vi "Migrate G Plug-in.vi"() -> ()   [LabVIEW 2021]
uses:
  _Measurement Migrator/Migrator/Queue Driver/controls/Queue Operations.ctl
  _Measurement Migrator/Migrator/Migration Logic/controls/Multiple Migration/Multiple Migration Data Holder.ctl
  <vilib>/Utility/sysdir.llb/System Directory Type.ctl
  <vilib>/Utility/miscctls.llb/LVRowAndColumnUnsignedTypeDef.ctl
  <vilib>/Utility/miscctls.llb/LVRowAndColumnTypeDef.ctl
  _Measurement Migrator/Migrator/Migrator Reusables/controls/Dictionary States.ctl
  <vilib>/Utility/cursorutil.llb/Set Cursor (Icon Pict).vi
  _Measurement Migrator/Migrator/Queue Driver/Queue Driver.lvlib
  _Measurement Migrator/Migrator/Migration Logic/Migrator.lvlib
  _Measurement Migrator/Migrator/Path Functions/Path Functions.lvlib
  _Measurement Migrator/Migrator/Multiple Migrator/Multiple Migrator.lvlib
  _Measurement Migrator/Migrator/Migrator Reusables/Migrator Reusables.lvlib
  _Measurement Migrator/Migrator/G Plug-in Migrator/G Plug-in Migrator.lvlib
panel:
  out "error out":errorcluster
  in  "Tab Control":T1(tab)
  in  "Info":string
  in  "Select Measurement":path
  out "Warning":bool=TRUE caption="Warning:\nSelected folder contains invalid folder/file names"
  in  "Populate measurements":bool
  in  "Select Project":path
  in  "Select all":bool
  in  "Back to Home":bool
  in  "List Plug-ins":bool
  in  "Select Measurements":string(tree)
  out "Selection warning":string="Atleast one measurement should be selected"
  out "Plug-in info":string="* Rename the Plug-in if required"
  out "Plug-in warning":string="Warning:\n1. Measurement plug-in name must be unique \n2. Plugin name cannot contain any of the following characters:\n         \\ / : * ? \" < > |"
  in  "Start Migration":bool
  in  "Back to Select":bool
  in  "List of Selected Measurements":i32(listbox)
  in  "Measurement Count":i32(slide)=6 caption="Migrating 2 of 2 measurement(s)" scale=0.0..100.0
  in  "Progress":i32(slide)=9 caption="Saving the project files..." scale=0.0..15.0
  in  "Review":bool
  in  "Migration Status":i32(listbox)
  in  "Back to Status":bool
  in  "Select Plug-in":string(combo) caption="Select Measurement plug-in to review"
  in  "Start Next":bool
  out "Launch Type Spec":string
  out "Launch Logic":string
  out "Launch UI":string
  # "* Project in which the measurement plug-in will be created"
  # "* Select a measurement vi or a folder containing measurements"
  # ".lvproj"
  # "Select the measurements to migrate"
  # "Review the Measurement:\n1. Review the Measurement UI. Click here to launch.\n2. Review the Measurement Logic VI. Click here to launch.\n3. Review the Type Specialization VI. Click here to launch."
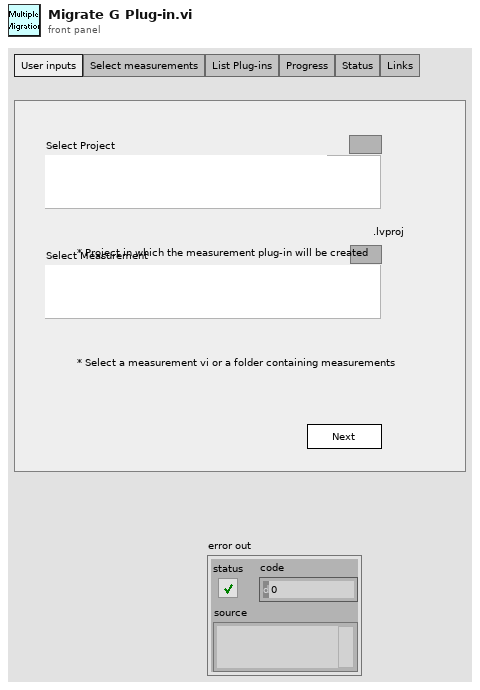
[diagram p1: front panel]
types:
  T1 = enum32{"User inputs", "Select measurements", "List Plug-ins", "Progress", "Status", "Links"}
  T2 = typedef "Queue Driver.lvlib/Queue Operations.ctl" = enum16{"Create Q", "Enqueue", "Enqueue N", "Dequeue", "Flush", "Release"}
  T3 = typedef "Migrator.lvlib/Multiple Migration Data Holder.ctl" = cluster{"Tree Reference":refnum<vi>, "LabVIEW Version":string, "Project path":path, "Create new project?":bool, "Measurement file/folder path":path, "Measurement folder selected?":bool, "Project warning":string, "Measurement warning":string, "Next clicked?":bool, "Measurement path changed?":bool, "Select all":bool, "Measurement folder Tags":string[], "Measurement file Tags":string[], "Selected cell Tag":string, "Measurement Plug-ins":string[][], "Measurement File Paths":path[], "Plugin Migration Value":i32, "Migration Count":i32, "Instrument containing subVIs":path[][], "Progress per measurement":i32, "Measurement Progress":i32, "Migration Status":string[][], "Selected Measurement":string[]}
  T4 = enum8{"Enabled", "Disabled", "Disabled and Grayed Out"}
  T5 = typedef "LVRowAndColumnUnsignedTypeDef.ctl" = cluster{"Row":u32, "Column":u32}
  T6 = typedef "LVRowAndColumnTypeDef.ctl" = cluster{"Row":i32, "Column":i32}
  T7 = typedef "Migrator Reusables.lvlib/Dictionary States.ctl" = enum16{"Set", "Get", "Delete", "Delete All"}
  T8 = typedef "System Directory Type.ctl" = i32
  T9 = typedef "LVPoint32TypeDef.ctl" = cluster{"Horizontal":i32, "Vertical":i32}
  T10 = typedef "Migrator.lvlib/Tree Items.ctl" = cluster{"Item name":string, "Indent":i32, "Tag":string}
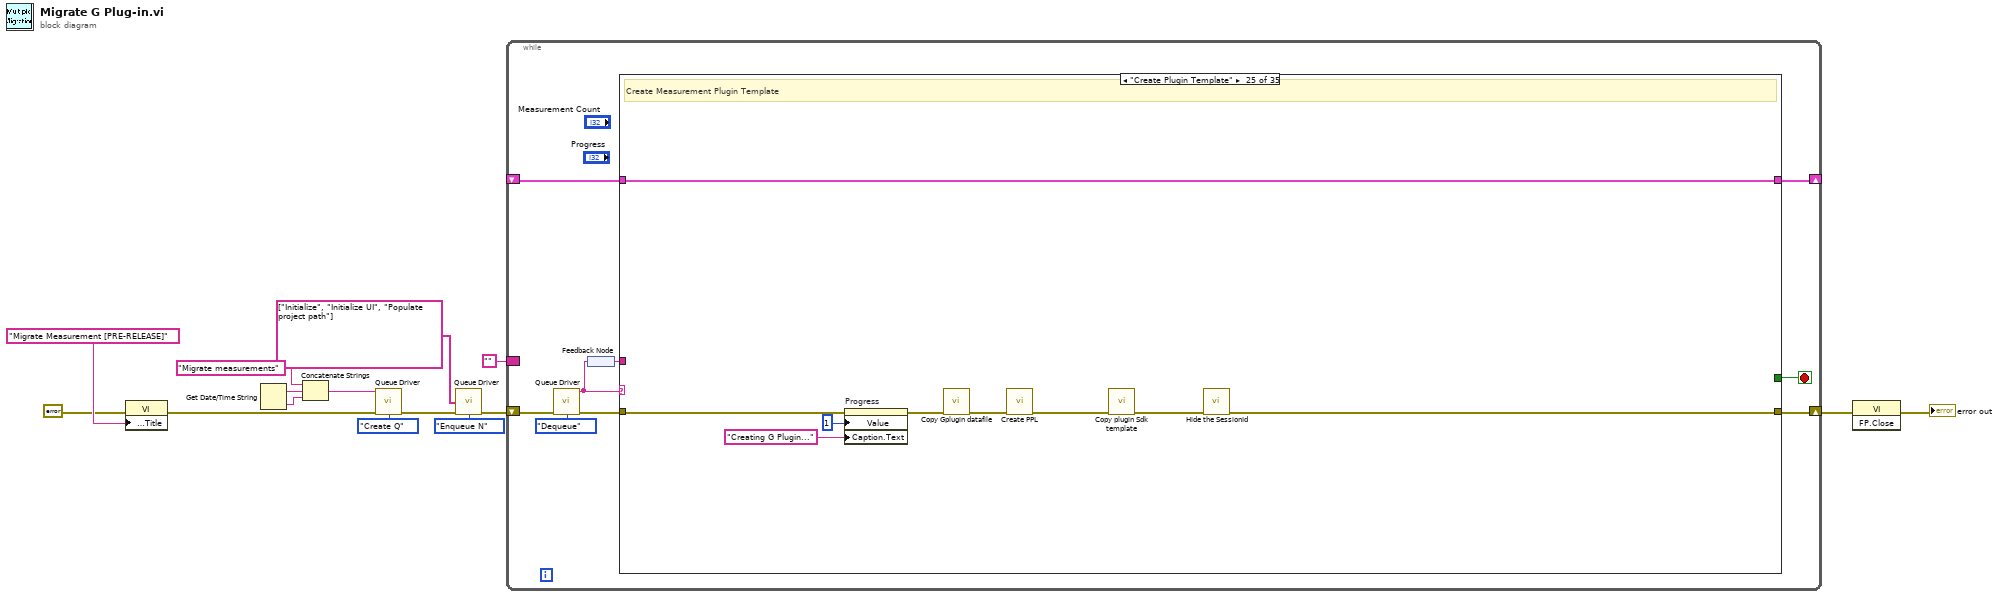
[diagram p0: block diagram]
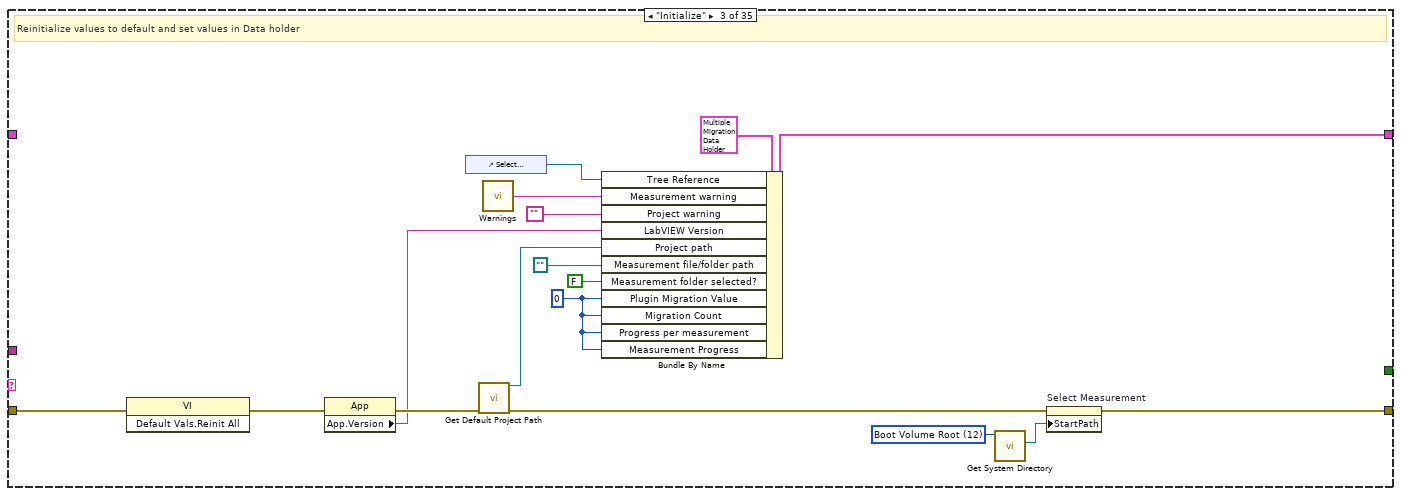
[diagram p4: hidden frame]
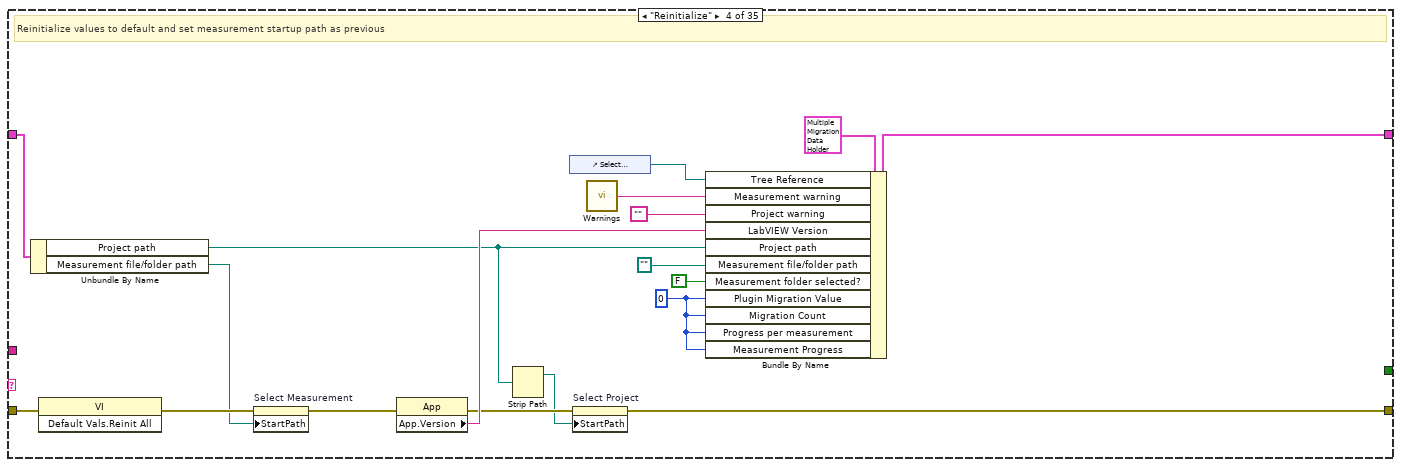
[diagram p5: hidden frame]
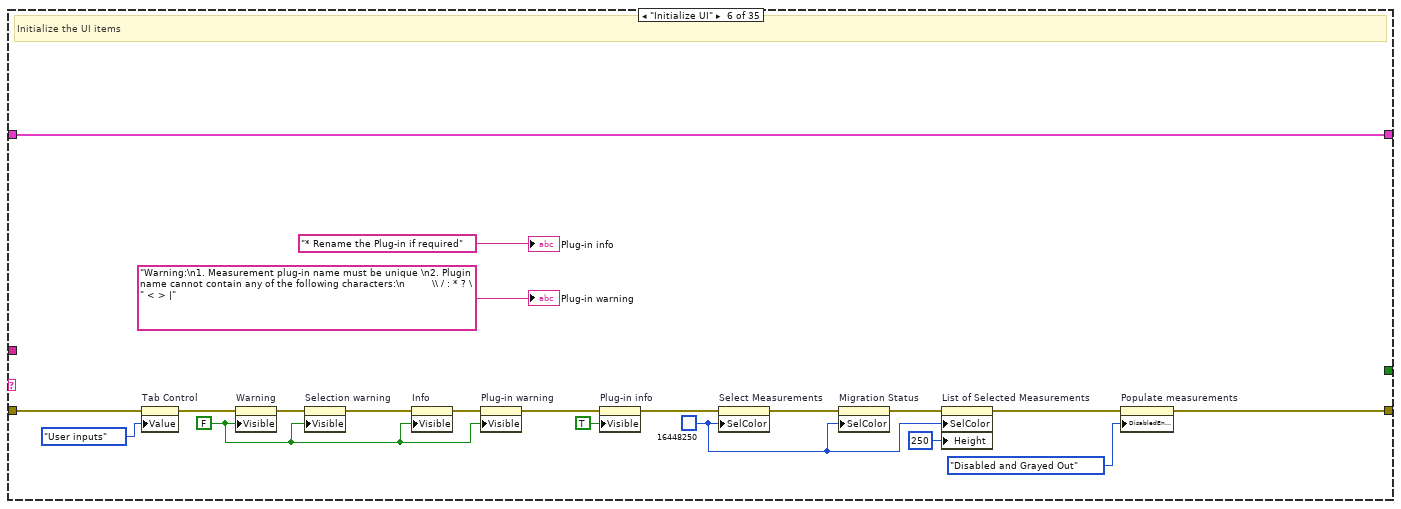
[diagram p7: hidden frame]
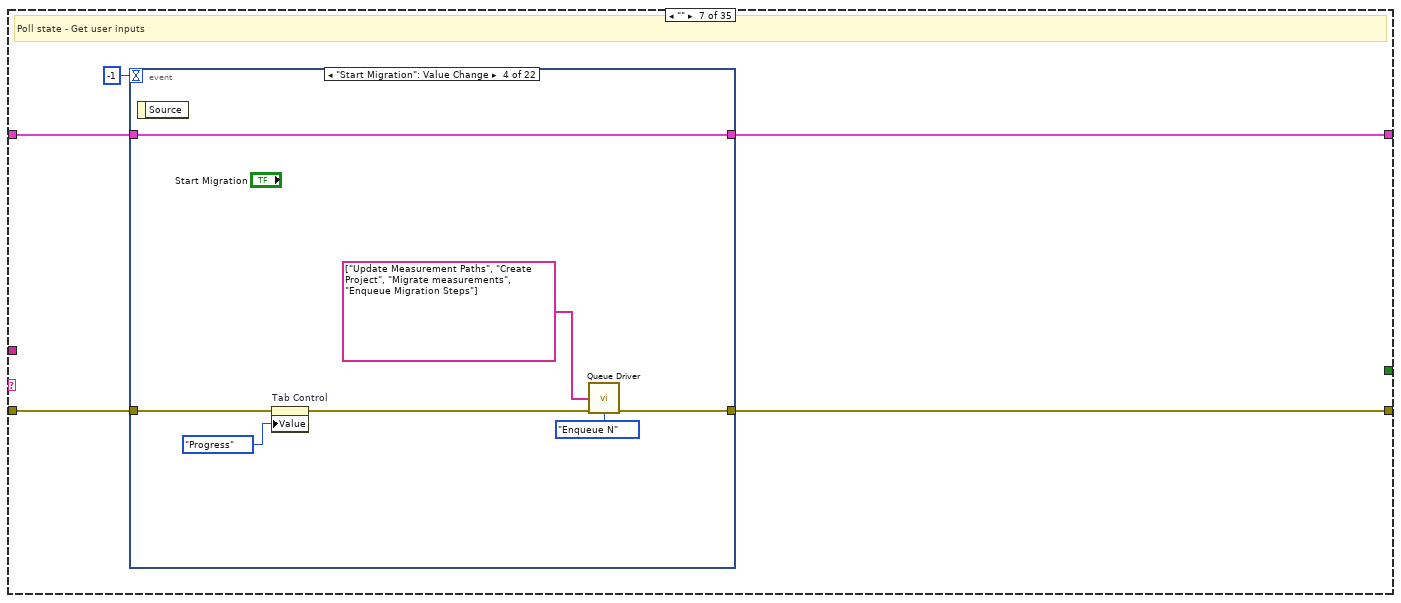
[diagram p8: hidden frame]
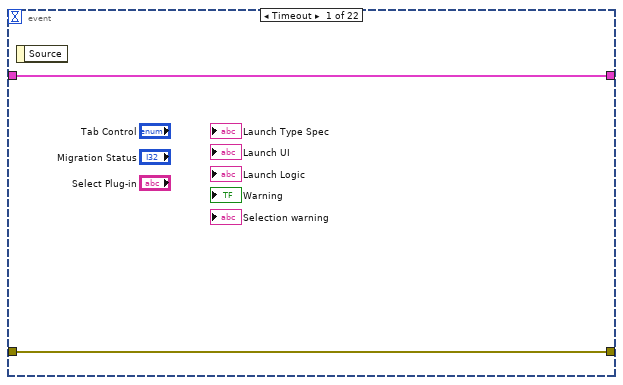
[diagram p9: hidden frame]
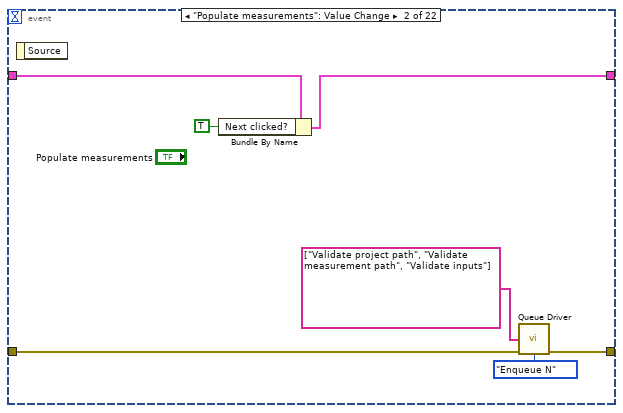
[diagram p10: hidden frame]
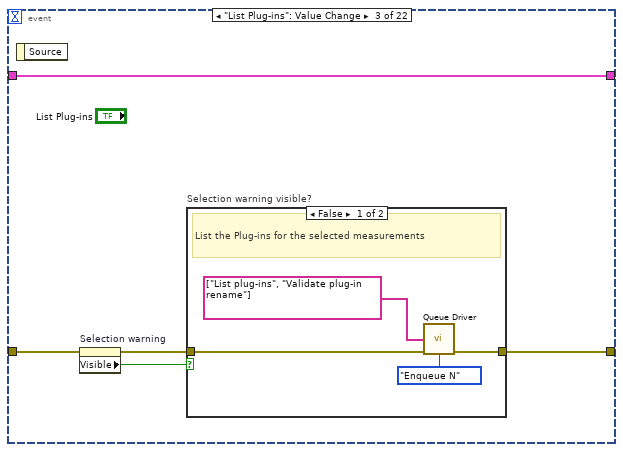
[diagram p11: hidden frame]
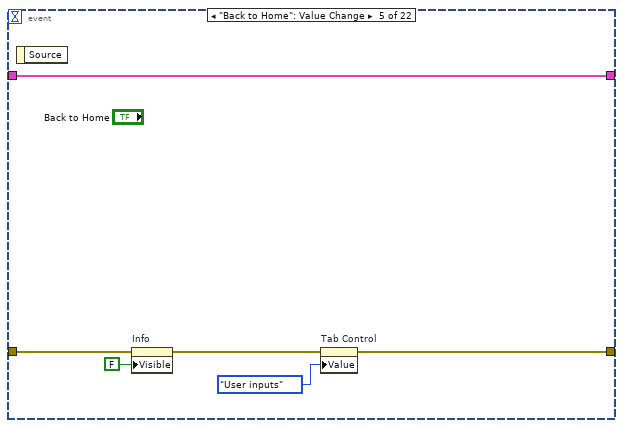
[diagram p13: hidden frame]
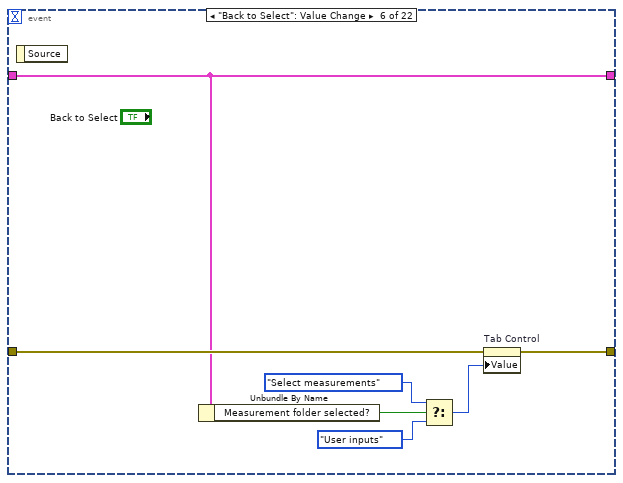
[diagram p14: hidden frame]
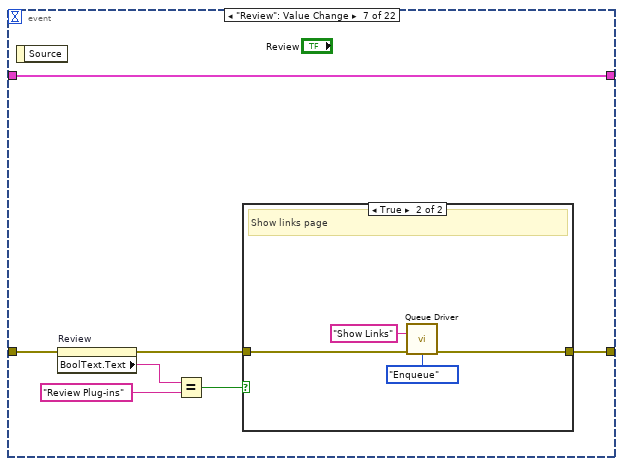
[diagram p15: hidden frame]
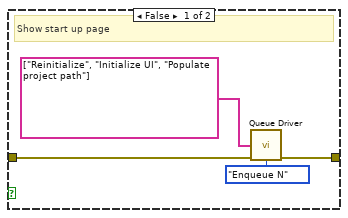
[diagram p16: hidden frame]
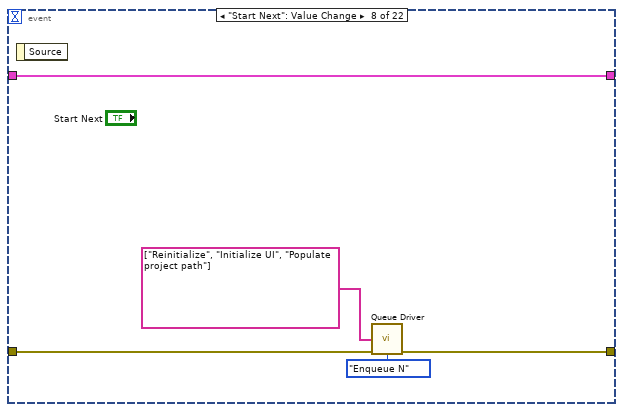
[diagram p17: hidden frame]
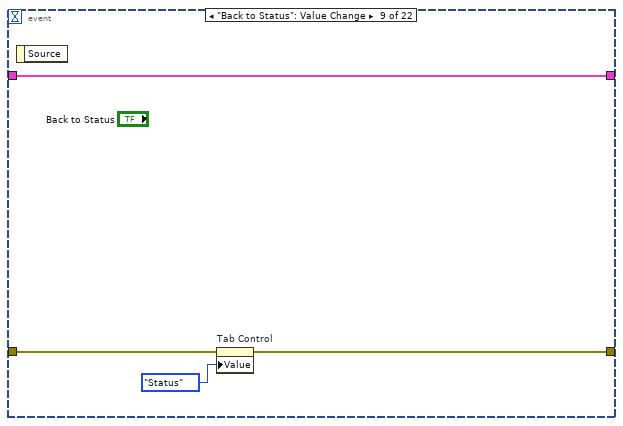
[diagram p18: hidden frame]
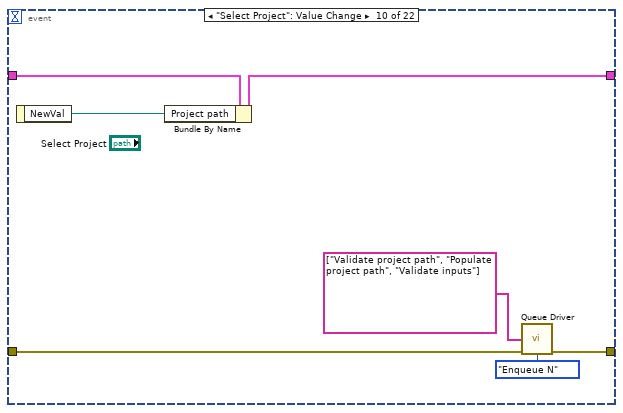
[diagram p19: hidden frame]
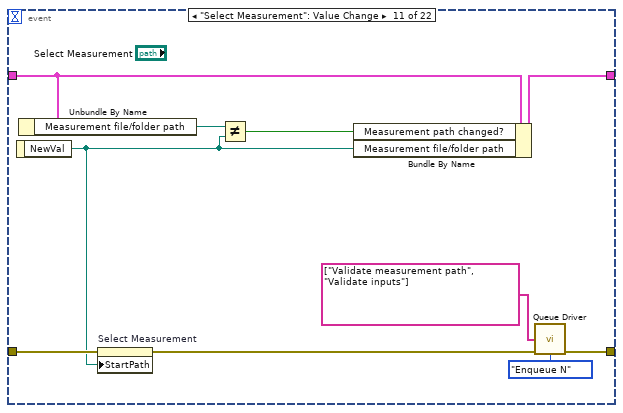
[diagram p20: hidden frame]
diagram:
  n1 = property class="VI"(error in=errorcluster {"status"=FALSE, "code"=0, "source"=""} ("error in (no error)"), "Front Panel.Title"="Migrate Measurement [PRE-RELEASE]" ("Front Panel Window:Title")) -> (error out=w1:errorcluster)  [unwired: 1 in, 1 out]
  n2 = Get Date/Time String() -> (date string=w12:string, time string=w11:string)  [unwired: 3 in]
  n3 = Concatenate Strings("Migrate measurements" ("string"), w12, w11) -> (w7:string)
  n4 = call "Queue Driver.vi"("Name"=w7, "error in (no error)"=w1, "Q Operations"=Queue_Operations."Create Q") -> ("error out"=w15:errorcluster)  [unwired: 11 in, 1 out]
  n5 = call "Queue Driver.vi"("States[]"=string[] ["Initialize", "Initialize UI", "Populate project path"], "error in (no error)"=w15, "Q Operations"=Queue_Operations."Enqueue N") -> ("error out"=w10:errorcluster)  [unwired: 11 in, 1 out]
  n6 = while {
    shift-right: [w23] -> w6
    shift-left: w10 -> [w24]
    shift-right: [w20] -> _
    shift-left: _ -> [w19]
    border: "" -> [_]
    stop <- w18 stop-if-true
    n7 = call "Queue Driver.vi"("error in (no error)"=w24, "Q Operations"=Queue_Operations."Dequeue") -> ("Dequeued State"=w17:string, "error out"=w22:errorcluster)  [unwired: 12 in]
    n8 = feedback #1() -> (w16:string)
    n9 = feedback-in #1(w17) -> ()
    n10 = case shown="\"Create Plugin Template\"" w17 {
      tunnel: w22 -> [w25 w28 w45 w63 w65 w85 w90 w265 w277 w288 w307 w331 w376 w393 w446 w471 w492 w549 w559 w566 w586 w596 w615 w632 w658 w662 w668 w690 w711 w723 w765 w774 w783 w804 w816]
      tunnel: [w25 w28 w34 w48 w65 w76 w89 w267 w277 w280 w306 w330 w376 w388 w434 w454 w479 w539 w559 w561 w583 w599 w614 w631 w653 w663 w672 w694 w711 w722 w762 w774 w780 w804 w806] -> w23
      tunnel: [w26 w27 w44 w62 w64 w81 w86 w266 w278 w283 w300 w318 w377 w394 w437 w469 w476 w544 w558 w578 w594 w608 w618 w651 w660 w666 w673 w695 w712 w727 w764 w775 w785 w805 w814] -> w20
      tunnel: w19 -> [w26 w27 _ w51 w64 w81 w87 w266 w278 w284 w302 w329 w377 w395 w438 w470 w477 w545 w558 w579 w594 w607 w618 w651 w660 w666 w674 w696 w712 w728 w764 w775 w785 w805 w814]
      tunnel: [_ _ _ _ _ _ _ _ _ _ _ _ _ _ _ _ _ _ _ _ _ _ _ _ _ _ _ _ _ _ _ _ _ _ TRUE] -> w18
      tunnel: w16 -> [_ _ _ _ _ _ _ _ _ _ _ _ _ _ _ _ _ _ _ _ _ _ _ _ _ _ _ _ _ _ _ _ w776 _ _]
      frame Default {
        # "Default case"
      }
      frame "/**********INITIALIZE**********/" {
      }
      frame "Initialize" {
        w29 = 0 ("Plugin Migration Value")
        w33 = T8 12 items=["User Home"=0, "User Desktop"=1, "User Documents"=2, "User Application Data"=3, "User Preferences"=4, "User Temporary"=5, "Public Documents"=6, "Public Application Data"=7, "Public Preferences"=8, "Public Cache"=13, "System Core Libraries"=9, "System Installed Libraries"=10, "Application Files"=11, "Boot Volume Root"=12] ("system directory type")
        # "Reinitialize values to default and set values in Data holder"
        n11 = invoke class="VI" method="Default Vals.Reinit All"(error in=w45) -> (error out=w42:errorcluster)  [unwired: 2 in, 2 out]
        n12 = property class="App"(error in=w42) -> (error out=w41:errorcluster, "App.Version"=w40:string)  [unwired: 1 in, 1 out]
        n13 = control-ref of="Select Measurements"() -> (w37:refnum<vi>)
        n14 = call "Get Default Project Path.vi"("error in"=w41) -> ("Project Path"=w43:path, "error out"=w35:errorcluster)  [unwired: 13 in]
        n15 = call "Warnings.vi"() -> ("Invalid measurement path"=w36:string)  [unwired: 8 in, 7 out]
        n16 = Bundle By Name(cluster=T3 {"Tree Reference"=refnum, "LabVIEW Version"="", "Project path"=path "", "Create new project?"=FALSE, "Measurement file/folder path"=path "", "Measurement folder selected?"=FALSE, "Project warning"="", "Measurement warning"="", "Next clicked?"=FALSE, "Measurement path changed?"=FALSE, "Select all"=FALSE, "Measurement folder Tags"=[], "Measurement file Tags"=[], "Selected cell Tag"="", "Measurement Plug-ins"=[], "Measurement File Paths"=[], "Plugin Migration Value"=0, "Migration Count"=0, "Instrument containing subVIs"=[], "Progress per measurement"=0, "Measurement Progress"=0, "Migration Status"=[], "Selected Measurement"=[]}, "Tree Reference"=w37, "Measurement warning"=w36, "Project warning"="", "LabVIEW Version"=w40, "Project path"=w43, "Measurement file/folder path"=path "", "Measurement folder selected?"=FALSE, "Plugin Migration Value"=w29, "Migration Count"=w29, "Progress per measurement"=w29, "Measurement Progress"=w29) -> (w44:T3)
        n17 = call <vilib>:"Get System Directory.vi"("system directory type"=w33) -> ("system directory"=w32:path)  [unwired: 10 in]
        n18 = property on="Select Measurement" class="Path"(error in=w35, "StartPath"=w32) -> (error out=w34:errorcluster)  [unwired: 1 in, 1 out]
      }
      frame "Reinitialize" {
        w54 = 0 ("Plugin Migration Value")
        # "Reinitialize values to default and set measurement startup path as previous"
        n19 = Unbundle By Name(w51) -> ("Project path"=w47:path, "Measurement file/folder path"=w50:path)
        n20 = invoke class="VI" method="Default Vals.Reinit All"(error in=w63) -> (error out=w53:errorcluster)  [unwired: 2 in, 2 out]
        n21 = property on="Select Measurement" class="Path"(error in=w53, "StartPath"=w50) -> (error out=w52:errorcluster)  [unwired: 1 in, 1 out]
        n22 = property class="App"(error in=w52) -> (error out=w49:errorcluster, "App.Version"=w61:string)  [unwired: 1 in, 1 out]
        n23 = Strip Path(path=w47) -> (stripped path=w46:path)  [unwired: 1 out]
        n24 = control-ref of="Select Measurements"() -> (w58:refnum<vi>)
        n25 = property on="Select Project" class="Path"(error in=w49, "StartPath"=w46) -> (error out=w48:errorcluster)  [unwired: 1 in, 1 out]
        n26 = call "Warnings.vi"() -> ("Invalid measurement path"=w57:string)  [unwired: 8 in, 7 out]
        n27 = Bundle By Name(cluster=T3 {"Tree Reference"=refnum, "LabVIEW Version"="", "Project path"=path "", "Create new project?"=FALSE, "Measurement file/folder path"=path "", "Measurement folder selected?"=FALSE, "Project warning"="", "Measurement warning"="", "Next clicked?"=FALSE, "Measurement path changed?"=FALSE, "Select all"=FALSE, "Measurement folder Tags"=[], "Measurement file Tags"=[], "Selected cell Tag"="", "Measurement Plug-ins"=[], "Measurement File Paths"=[], "Plugin Migration Value"=0, "Migration Count"=0, "Instrument containing subVIs"=[], "Progress per measurement"=0, "Measurement Progress"=0, "Migration Status"=[], "Selected Measurement"=[]}, "Tree Reference"=w58, "Measurement warning"=w57, "Project warning"="", "LabVIEW Version"=w61, "Project path"=w47, "Measurement file/folder path"=path "", "Measurement folder selected?"=FALSE, "Plugin Migration Value"=w54, "Migration Count"=w54, "Progress per measurement"=w54, "Measurement Progress"=w54) -> (w62:T3)
      }
      frame "/**********FP RELATED**********/" {
      }
      frame "Initialize UI" {
        w70 = FALSE ("Visible")
        w78 = u32 16448250 ("Selection Color")
        # "Initialize the UI items"
        n28 = property on="Tab Control" class="TabCtl (strict)"(error in=w85, "Value"=T1."User inputs" ("Tab Control")) -> (error out=w80:errorcluster)  [unwired: 1 in, 1 out]
        n29 = property on="Warning" class="Bool"(error in=w80, "Visible"=w70) -> (error out=w79:errorcluster)  [unwired: 1 in, 1 out]
        n30 = property on="Selection warning" class="Str"(error in=w79, "Visible"=w70) -> (error out=w74:errorcluster)  [unwired: 1 in, 1 out]
        n31 = property on="Info" class="Str"(error in=w74, "Visible"=w70) -> (error out=w73:errorcluster)  [unwired: 1 in, 1 out]
        n32 = property on="Plug-in warning" class="Str"(error in=w73, "Visible"=w70) -> (error out=w69:errorcluster)  [unwired: 1 in, 1 out]
        n33 = property on="Plug-in info" class="Str"(error in=w69, "Visible"=TRUE) -> (error out=w68:errorcluster)  [unwired: 1 in, 1 out]
        n34 = property on="Select Measurements" class="Tree (strict)"(error in=w68, "SelColor"=w78) -> (error out=w83:errorcluster)  [unwired: 1 in, 1 out]
        n35 = property on="Migration Status" class="MCListbox (strict)"(error in=w83, "SelColor"=w78) -> (error out=w82:errorcluster)  [unwired: 1 in, 1 out]
        n36 = property on="List of Selected Measurements" class="MCListbox (strict)"(error in=w82, "SelColor"=w78, "Height"=u32 250 ("Size:Height")) -> (error out=w77:errorcluster)  [unwired: 1 in, 1 out]
        n37 = property on="Populate measurements" class="Bool"(error in=w77, "DisabledEnum"=T4."Disabled and Grayed Out" ("Disabled")) -> (error out=w76:errorcluster)  [unwired: 1 in, 1 out]
        "Plug-in warning" <- "Warning:\n1. Measurement plug-in name must be unique \n2. Plugin name cannot contain any of the following characters:\n         \\ / : * ? \" < > |" ("f")
        "Plug-in info" <- "* Rename the Plug-in if required" ("Plug-in warning")
      }
      frame "" {
        # "Poll state - Get user inputs"
        n38 = event shown="[3] \"Start Migration\": Value Change" {
          selector: _ -> [_ _ _ _ _ _ _ _ _ _ _ _ _ _ _ _ _ _ _ _ _ _]
          dyn-events: _ -> [_ _ _ _ _ _ _ _ _ _ _ _ _ _ _ _ _ _ _ _ _ _]
          timeout: -1 -> [_ _ _ _ _ _ _ _ _ _ _ _ _ _ _ _ _ _ _ _ _ _]
          tunnel: w90 -> [w92 w99 w102 w116 w119 w129 w133 w146 w153 w160 w166 w174 w185 w192 w205 w212 w215 w219 w225 w235 w247 w259]
          tunnel: [w92 w98 w103 w112 w122 w128 w135 w147 w152 w159 w169 w173 w180 w191 w203 w213 w216 w220 w227 w238 w249 w258] -> w89
          tunnel: w87 -> [w91 w95 w104 w113 w120 w127 w136 w149 w150 w157 w164 w177 w184 w193 w206 w214 w218 w222 w228 w239 w250 w260]
          tunnel: [w91 w94 w104 w113 w120 w127 w136 w149 w150 w156 w170 w176 w183 w193 w206 w214 w218 w222 w228 w239 w250 w260] -> w86
          event Timeout {
            # "Timeout"
            n39 = event-data() -> ()  [unwired: 1 in, 1 out]
          }
          event "Populate measurements": Value Change {
            n40 = event-data() -> ()  [unwired: 1 in, 1 out]
            n41 = Bundle By Name(cluster=w95, "Next clicked?"=TRUE) -> (w94:T3)
            n42 = call "Queue Driver.vi"("States[]"=string[] ["Validate project path", "Validate measurement path", "Validate inputs"], "error in (no error)"=w99, "Q Operations"=Queue_Operations."Enqueue N") -> ("error out"=w98:errorcluster)  [unwired: 11 in, 1 out]
          }
          event "List Plug-ins": Value Change {
            n43 = event-data() -> ()  [unwired: 1 in, 1 out]
            n44 = property on="Selection warning" class="Str"(error in=w102) -> (error out=w101:errorcluster, "Visible"=w100:bool)  [unwired: 1 in, 1 out]
            n45 = case "Selection warning visible?" shown="False" w100 {
              tunnel: w101 -> [w108 w109]
              tunnel: [w107 w109] -> w103
              frame False {
                # "List the Plug-ins for the selected measurements"
                n46 = call "Queue Driver.vi"("States[]"=string[] ["List plug-ins", "Validate plug-in rename"], "error in (no error)"=w108, "Q Operations"=Queue_Operations."Enqueue N") -> ("error out"=w107:errorcluster)  [unwired: 11 in, 1 out]
              }
              frame True {
                # "Pass"
              }
            }
          }
          event "Start Migration": Value Change {
            n47 = event-data() -> ()  [unwired: 1 in, 1 out]
            n48 = property on="Tab Control" class="TabCtl (strict)"(error in=w116, "Value"=T1."Progress" ("Tab Control")) -> (error out=w115:errorcluster)  [unwired: 1 in, 1 out]
            n49 = call "Queue Driver.vi"("States[]"=string[] ["Update Measurement Paths", "Create Project", "Migrate measurements", "Enqueue Migration Steps"], "error in (no error)"=w115, "Q Operations"=Queue_Operations."Enqueue N") -> ("error out"=w112:errorcluster)  [unwired: 11 in, 1 out]
          }
          event "Back to Home": Value Change {
            n50 = event-data() -> ()  [unwired: 1 in, 1 out]
            n51 = property on="Info" class="Str"(error in=w119, "Visible"=FALSE) -> (error out=w118:errorcluster)  [unwired: 1 in, 1 out]
            n52 = property on="Tab Control" class="TabCtl (strict)"(error in=w118, "Value"=T1."User inputs" ("Tab Control")) -> (error out=w122:errorcluster)  [unwired: 1 in, 1 out]
          }
          event "Back to Select": Value Change {
            n53 = event-data() -> ()  [unwired: 1 in, 1 out]
            n54 = Unbundle By Name(w127) -> ("Measurement folder selected?"=w126:bool)
            n55 = Select(t=T1."Select measurements" ("Tab Control"), s=w126, f=T1."User inputs" ("Tab Control")) -> (s? t:f=w123:T1)
            n56 = property on="Tab Control" class="TabCtl (strict)"(error in=w129, "Value"=w123) -> (error out=w128:errorcluster)  [unwired: 1 in, 1 out]
          }
          event "Review": Value Change {
            n57 = event-data() -> ()  [unwired: 1 in, 1 out]
            n58 = property on="Review" class="Bool"(error in=w133) -> (error out=w134:errorcluster, "BoolText.Text"=w132:string)  [unwired: 1 in, 1 out]
            n59 = Equal?(x=w132, y="Review Plug-ins") -> (x = y?=w130:bool)
            n60 = case shown="True" w130 {
              tunnel: [w138 w144] -> w135
              tunnel: w134 -> [w137 w141]
              frame False {
                # "Show start up page"
                n61 = call "Queue Driver.vi"("States[]"=string[] ["Reinitialize", "Initialize UI", "Populate project path"], "error in (no error)"=w137, "Q Operations"=Queue_Operations."Enqueue N") -> ("error out"=w138:errorcluster)  [unwired: 11 in, 1 out]
              }
              frame True {
                # "Show links page"
                n62 = call "Queue Driver.vi"("State"="Show Links", "error in (no error)"=w141, "Q Operations"=Queue_Operations."Enqueue") -> ("error out"=w144:errorcluster)  [unwired: 11 in, 1 out]
              }
            }
          }
          event "Start Next": Value Change {
            n63 = event-data() -> ()  [unwired: 1 in, 1 out]
            n64 = call "Queue Driver.vi"("States[]"=string[] ["Reinitialize", "Initialize UI", "Populate project path"], "error in (no error)"=w146, "Q Operations"=Queue_Operations."Enqueue N") -> ("error out"=w147:errorcluster)  [unwired: 11 in, 1 out]
          }
          event "Back to Status": Value Change {
            n65 = event-data() -> ()  [unwired: 1 in, 1 out]
            n66 = property on="Tab Control" class="TabCtl (strict)"(error in=w153, "Value"=T1."Status" ("Tab Control")) -> (error out=w152:errorcluster)  [unwired: 1 in, 1 out]
          }
          event "Select Project": Value Change {
            n67 = event-data() -> ("NewVal"=w155:path)  [unwired: 1 in]
            n68 = Bundle By Name(cluster=w157, "Project path"=w155) -> (w156:T3)
            n69 = call "Queue Driver.vi"("States[]"=string[] ["Validate project path", "Populate project path", "Validate inputs"], "error in (no error)"=w160, "Q Operations"=Queue_Operations."Enqueue N") -> ("error out"=w159:errorcluster)  [unwired: 11 in, 1 out]
          }
          event "Select Measurement": Value Change {
            n70 = event-data() -> ("NewVal"=w161:path)  [unwired: 1 in]
            n71 = Unbundle By Name(w164) -> ("Measurement file/folder path"=w162:path)
            n72 = property on="Select Measurement" class="Path"(error in=w166, "StartPath"=w161) -> (error out=w165:errorcluster)  [unwired: 1 in, 1 out]
            n73 = Not Equal?(x=w162, y=w161) -> (x != y?=w163:bool)
            n74 = Bundle By Name(cluster=w164, "Measurement path changed?"=w163, "Measurement file/folder path"=w161) -> (w170:T3)
            n75 = call "Queue Driver.vi"("States[]"=string[] ["Validate measurement path", "Validate inputs"], "error in (no error)"=w165, "Q Operations"=Queue_Operations."Enqueue N") -> ("error out"=w169:errorcluster)  [unwired: 11 in, 1 out]
          }
          event "Select all": Value Change {
            n76 = event-data() -> ("NewVal"=w175:bool)  [unwired: 1 in]
            n77 = Bundle By Name(cluster=w177, "Select all"=w175) -> (w176:T3)
            n78 = call "Queue Driver.vi"("State"="Select/Deselect all", "error in (no error)"=w174, "Q Operations"=Queue_Operations."Enqueue") -> ("error out"=w173:errorcluster)  [unwired: 11 in, 1 out]
          }
          event "Select Measurements": Mouse Down {
            n79 = event-data() -> ("Coords"=w178:T9)  [unwired: 1 in]
            n80 = invoke on="Select Measurements" class="Tree (strict)" method="Point To Row Column"(error in=w185, "Point"=w178) -> (error out=w181:errorcluster, "Tag"=w182:string, "InGlyph"=w179:bool)  [unwired: 6 in, 5 out]
            n81 = case "In Symbol?" shown="True" w179 {
              tunnel: w181 -> [w186 w190]
              tunnel: [w186 w189] -> w180
              frame False {
                # "Pass"
              }
              frame True {
                # "Update the selection of measurements"
                n82 = call "Queue Driver.vi"("State"="Measurement selection" ("State 2"), "error in (no error)"=w190, "Q Operations"=Queue_Operations."Enqueue") -> ("error out"=w189:errorcluster)  [unwired: 11 in, 1 out]
              }
            }
            n83 = Bundle By Name(cluster=w184, "Selected cell Tag"=w182) -> (w183:T3)
          }
          event "List of Selected Measurements": Edit Cell {
            n84 = event-data() -> ()  [unwired: 1 in, 1 out]
            n85 = disable-structure shown="Enabled" {
              disable-tunnel: w192 -> [w197 w198]
              disable-tunnel: [w196 w198] -> w191
              frame Disabled {
                n86 = call "Queue Driver.vi"("State"="Validate plug-in rename", "error in (no error)"=w197, "Q Operations"=Queue_Operations."Enqueue") -> ("error out"=w196:errorcluster)  [unwired: 11 in, 1 out]
              }
              frame Enabled {
              }
            }
          }
          event "List of Selected Measurements": Mouse Down {
            n87 = event-data() -> ("Coords"=w202:T9)  [unwired: 1 in, 7 out]
            n88 = invoke on="List of Selected Measurements" class="MCListbox (strict)" method="Point To Row Column"(error in=w205, "Point"=w202) -> (error out=w204:errorcluster, "CellPosition"=w199:T6)  [unwired: 5 in, 5 out]
            n89 = Unbundle By Name(w199) -> ("Column"=w201:i32)
            n90 = Not Equal To 0?(x=w201) -> (x != 0?=w200:bool)
            n91 = case shown="True" w200 {
              tunnel: w204 -> [w207 w210]
              tunnel: [w207 w209] -> w203
              tunnel: w199 -> [_ w208]
              frame False {
              }
              frame True {
                n92 = property on="List of Selected Measurements" class="MCListbox (strict)"(error in=w210, "EditPos"=w208) -> (error out=w209:errorcluster)  [unwired: 1 in, 1 out]
              }
            }
          }
          event "Select Plug-in": Value Change {
            n93 = event-data() -> ("NewVal"=w211:string)  [unwired: 1 in]
            n94 = call "Set Measurement Name.vi"("Name"=w211, "error in (no error)"=w212) -> ("error out"=w213:errorcluster)  [unwired: 13 in]
          }
          event "Launch UI", "Launch Logic", "Launch Type Spec": Mouse Enter {
            n95 = event-data() -> ()  [unwired: 1 in, 1 out]
            n96 = call-poly <vilib>:"Set Cursor.vi"("error in (no error)"=w215, "icon"=u16 6) -> ("error out"=w216:errorcluster)  [unwired: 8 in, 1 out]
          }
          event "Launch UI", "Launch Logic", "Launch Type Spec": Mouse Leave {
            n97 = event-data() -> ()  [unwired: 1 in, 1 out]
            n98 = call-poly <vilib>:"Set Cursor.vi"("error in (no error)"=w219, "icon"=u16 0) -> ("error out"=w220:errorcluster)  [unwired: 8 in, 1 out]
          }
          event "Launch UI": Mouse Down {
            n99 = event-data() -> ()  [unwired: 1 in, 1 out]
            n100 = property on="Select Plug-in" class="CmbBox"(error in=w225) -> (error out=w226:errorcluster, "Value"=w224:string)  [unwired: 1 in, 1 out]
            n101 = Empty String/Path?(string/path=w224) -> (empty?=w223:bool)
            n102 = case shown="False" w223 {
              tunnel: [w231 w233] -> w227
              tunnel: w226 -> [w229 w233]
              frame False {
                n103 = call "Measurement Plugin Path.vi"("error in (no error)"=w229) -> ("Measurement UI"=w230:path, "error out"=w232:errorcluster)  [unwired: 2 in, 11 out]
                n104 = call "Open VI.vi"("Logic VI Path"=w230, "error in (no error)"=w232) -> ("error out"=w231:errorcluster)  [unwired: 13 in]
              }
              frame True {
              }
            }
          }
          event "Launch Logic": Mouse Down {
            n105 = event-data() -> ()  [unwired: 1 in, 1 out]
            n106 = property on="Select Plug-in" class="CmbBox"(error in=w235) -> (error out=w236:errorcluster, "Value"=w237:string)  [unwired: 1 in, 1 out]
            n107 = Empty String/Path?(string/path=w237) -> (empty?=w234:bool)
            n108 = case shown="False" w234 {
              tunnel: [w242 w244] -> w238
              tunnel: w236 -> [w241 w244]
              frame False {
                n109 = call "Measurement Plugin Path.vi"("error in (no error)"=w241) -> ("Logic VI Path"=w240:path, "error out"=w243:errorcluster)  [unwired: 2 in, 11 out]
                n110 = call "Open VI.vi"("Logic VI Path"=w240, "error in (no error)"=w243) -> ("error out"=w242:errorcluster)  [unwired: 13 in]
              }
              frame True {
              }
            }
          }
          event "Launch Type Spec": Mouse Down {
            n111 = event-data() -> ()  [unwired: 1 in, 1 out]
            n112 = property on="Select Plug-in" class="CmbBox"(error in=w247) -> (error out=w246:errorcluster, "Value"=w248:string)  [unwired: 1 in, 1 out]
            n113 = Empty String/Path?(string/path=w248) -> (empty?=w245:bool)
            n114 = case shown="False" w245 {
              tunnel: [w253 w255] -> w249
              tunnel: w246 -> [w252 w255]
              frame False {
                n115 = call "Measurement Plugin Path.vi"("error in (no error)"=w252) -> ("Type Specialization"=w251:path, "error out"=w254:errorcluster)  [unwired: 2 in, 11 out]
                n116 = call "Open VI.vi"("Logic VI Path"=w251, "error in (no error)"=w254) -> ("error out"=w253:errorcluster)  [unwired: 13 in]
              }
              frame True {
              }
            }
          }
          event Panel Close? {
            n117 = event-data() -> ()  [unwired: 1 in, 1 out]
            n118 = call "Queue Driver.vi"("State"="Exit", "error in (no error)"=w259, "Q Operations"=Queue_Operations."Enqueue") -> ("error out"=w258:errorcluster)  [unwired: 11 in, 1 out]
            n119 = event-data("Discard?"=TRUE) -> ()  [unwired: 1 in, 1 out]
          }
        }
      }
      frame "Populate project path" {
        # "Populate the validated project path in the control"
        n120 = Unbundle By Name(w266) -> ("Project warning"=w263:string, "Project path"=w264:path)
        n121 = Empty String/Path?(string/path=w263) -> (empty?=w262:bool)
        n122 = case "Valid project?" shown="True" w262 {
          tunnel: [w268 w276] -> w267
          tunnel: w265 -> [w268 w275]
          tunnel: w264 -> [_ w270]
          frame False {
            # "Pass"
          }
          frame True {
            # "Populate the path in the control"
            n123 = call <vilib>:"Get File Extension.vi"("error in (no error)"=w275, "file"=w270) -> ("error out"=w274:errorcluster, "filename without extension"=w273:string)  [unwired: 5 in, 3 out]
            n124 = Concatenate Strings("..\\" ("string"), w273) -> (w271:string)
            n125 = Build Path(base path=w270, name or relative path=w271) -> (appended path=w269:path)
            n126 = property on="Select Project" class="Path"(error in=w274, "Value"=w269) -> (error out=w276:errorcluster)  [unwired: 1 in, 1 out]
          }
        }
      }
      frame "/**********INPUT VALIDATION**********/" {
      }
      frame "Validate project path" {
        # "Validate the project path and set warning if required"
        n127 = Unbundle By Name(w284) -> ("Project path"=w285:path, "LabVIEW Version"=w286:string)
        n128 = call <vilib>:"Is Path and Not Empty.vi"("path"=w285) -> ("Is Path and Not Empty?"=w287:bool)  [unwired: 4 in]
        n129 = case "Is Path and not empty?" shown="True" w287 {
          tunnel: w288 -> [w291 w298]
          tunnel: [w291 w297] -> w280
          tunnel: [w289 w296] -> w279
          tunnel: w286 -> [_ w295]
          tunnel: w285 -> [w290 w294]
          tunnel: [_ w293] -> w282
          tunnel: [w290 w292] -> w281
          frame False {
            # "Set warning"
            n130 = call "Warnings.vi"() -> ("Invalid project path"=w289:string)  [unwired: 8 in, 7 out]
          }
          frame True {
            # "Validate the path"
            n131 = call "Validate Project Path.vi"("Project path in"=w294, "LabVIEW Version"=w295, "error in (no error)"=w298) -> ("Validated project path"=w292:path, "New project?"=w293:bool, "Warning"=w296:string, "error out"=w297:errorcluster)  [unwired: 9 in]
          }
        }
        n132 = Bundle By Name(cluster=w284, "Project path"=w281, "Create new project?"=w282, "Project warning"=w279) -> (w283:T3)
      }
      frame "Validate measurement path" {
        # "Validate the measurement path and set warning if required"
        n133 = Unbundle By Name(w302) -> ("Measurement file/folder path"=w304:path, "LabVIEW Version"=w305:string)
        n134 = call <vilib>:"Is Path and Not Empty.vi"("path"=w304) -> ("Is Path and Not Empty?"=w303:bool)  [unwired: 4 in]
        n135 = case "Is Path and not empty?" shown="True" w303 {
          tunnel: w307 -> [w309 w315]
          tunnel: w304 -> [_ w314]
          tunnel: w305 -> [_ w313]
          tunnel: [w309 w312] -> w306
          tunnel: [w308 w311] -> w299
          tunnel: [_ w310] -> w301
          frame False {
            # "Set warning"
            n136 = call "Warnings.vi"() -> ("Invalid measurement path"=w308:string)  [unwired: 8 in, 7 out]
          }
          frame True {
            # "Validate the path"
            n137 = call "Validate Measurement Path.vi"("Measurement path"=w314, "LabVIEW version"=w313, "error in (no error)"=w315) -> ("Folder?"=w310:bool, "Warning"=w311:string, "error out"=w312:errorcluster)  [unwired: 10 in]
          }
        }
        n138 = Bundle By Name(cluster=w302, "Measurement folder selected?"=w301, "Measurement warning"=w299) -> (w300:T3)
      }
      frame "Validate inputs" {
        # "Validate the project path and measurement path inputs"
        n139 = Unbundle By Name(w329) -> ("Project warning"=w323:string, "Measurement warning"=w328:string, "Next clicked?"=w324:bool, "Project warning"=w322:string, "Measurement warning"=w321:string, "Measurement folder selected?"=w320:bool, "Measurement path changed?"=w319:bool)
        n140 = Empty String/Path?(string/path=w328) -> (empty?=w327:bool)
        n141 = Empty String/Path?(string/path=w323) -> (empty?=w326:bool)
        n142 = And(x=w326, y=w327) -> (x .and. y?=w325:bool)
        n143 = case "Valid inputs?" shown="False" w325 {
          tunnel: w331 -> [w345 w355]
          tunnel: [w340 w351] -> w330
          tunnel: w324 -> [_ w349]
          tunnel: w322 -> [w333 _]
          tunnel: w321 -> [w336 _]
          tunnel: w320 -> [_ w348]
          tunnel: w319 -> [w332 w347]
          tunnel: [w332 w346] -> w316
          frame False {
            # "Set the appropriate warning"
            n144 = call "Edit Warning.vi"("Warning in"=w333) -> ("Warning out"=w335:string)  [unwired: 6 in]
            n145 = call "Edit Warning.vi"("Warning in"=w336) -> ("Warning out"=w334:string)  [unwired: 6 in]
            n146 = Concatenate Strings("Warning:" ("string"), "\n", w335, w334) -> (w338:string)
            n147 = call "Get Warning Position.vi"("Warning"=w338) -> ("Warning position"=w337:i32)  [unwired: 6 in]
            n148 = property on="Warning" class="Bool"(error in=w345, "Visible"=TRUE, "Caption.Text"=w338, "Caption.Top"=w337) -> (error out=w341:errorcluster)  [unwired: 1 in, 1 out]
            n149 = property on="Populate measurements" class="Bool"(error in=w341, "DisabledEnum"=T4."Disabled and Grayed Out" ("Disabled")) -> (error out=w340:errorcluster)  [unwired: 1 in, 1 out]
          }
          frame True {
            # "Check if next is clicked and make the warning invisible"
            n150 = case "Next clicked?" shown="True" w349 {
              tunnel: w355 -> [w357 w362]
              tunnel: [w357 w361] -> w354
              tunnel: w348 -> [_ w360]
              tunnel: w347 -> [w356 w359]
              tunnel: [w356 FALSE] -> w346
              frame False {
                # "Pass"
              }
              frame True {
                # "Populate measurements if folder is selected and List the plug-ins if not"
                n151 = case "Measurement path changed?" shown="True" w359 {
                  tunnel: w362 -> [w368 w375]
                  tunnel: [w367 w374] -> w361
                  tunnel: w360 -> [w363 w372]
                  frame False {
                    # "Measurement folder?"
                    n152 = Select(t=T1."Select measurements" ("Tab Control"), s=w363, f=T1."List Plug-ins" ("Tab Control")) -> (s? t:f=w364:T1)
                    n153 = property on="Tab Control" class="TabCtl (strict)"(error in=w368, "Value"=w364) -> (error out=w367:errorcluster)  [unwired: 1 in, 1 out]
                  }
                  frame True {
                    # "Measurement folder?"
                    n154 = Select(t=string[] ["Populate measurements"] ("States[]"), s=w372, f=string[] ["List plug-ins", "Validate plug-in rename"]) -> (s? t:f=w370:string[])
                    n155 = call "Queue Driver.vi"("States[]"=w370, "error in (no error)"=w375, "Q Operations"=Queue_Operations."Enqueue N") -> ("error out"=w374:errorcluster)  [unwired: 11 in, 1 out]
                  }
                }
              }
            }
            n156 = property on="Warning" class="Bool"(error in=w354, "Visible"=FALSE) -> (error out=w352:errorcluster)  [unwired: 1 in, 1 out]
            n157 = property on="Populate measurements" class="Bool"(error in=w352, "DisabledEnum"=T4."Enabled" ("Disabled")) -> (error out=w351:errorcluster)  [unwired: 1 in, 1 out]
          }
        }
        n158 = Bundle By Name(cluster=w329, "Next clicked?"=FALSE, "Measurement path changed?"=w316) -> (w318:T3)
      }
      frame "/**********FUNCTIONALITY**********/" {
      }
      frame "Populate measurements" {
        w382 = TRUE ("Visible")
        # "Populate the measurements in the Tree and set icon to the items"
        n159 = Unbundle By Name(w395) -> ("Tree Reference"=w389:refnum<vi>, "Measurement file/folder path"=w398:path, "LabVIEW Version"=w396:string)
        n160 = call "Set Cursor Icon.vi"("Cursor icon"=u16 2, "error in (no error)"=w393) -> ("error out"=w392:errorcluster)  [unwired: 13 in]
        n161 = property on="Info" class="Str"(error in=w392, "Visible"=w382, "Text.FontBold"=w382, "Text.Text"="Populating the measurements..." ("Info")) -> (error out=w391:errorcluster)  [unwired: 1 in, 1 out]
        n162 = call "Get Measurements.vi"("Input path"=w398, "LabVIEW version"=w396, "error in (no error)"=w391) -> ("Error?"=w383:string, "VI list"=w385:T10[], "Folder list"=w384:T10[], "error out"=w397:errorcluster)  [unwired: 9 in]
        n163 = Empty String/Path?(string/path=w383) -> (empty?=w386:bool)
        n164 = case "No error occured during get measurements?" shown="False" w386 {
          tunnel: w397 -> [w399 w431]
          tunnel: w395 -> [w406 w430]
          tunnel: [w405 w429] -> w394
          tunnel: w389 -> [w404 w428]
          tunnel: [w402 w427] -> w379
          tunnel: w385 -> [_ w418]
          tunnel: w384 -> [_ w417]
          tunnel: w383 -> [w403 _]
          frame False {
            # "Update the warning"
            n165 = Bundle By Name(cluster=w406, "Tree Reference"=w404, "Measurement warning"=w403) -> (w405:T3)
            n166 = call "Queue Driver.vi"("State"="Validate inputs", "error in (no error)"=w399, "Q Operations"=Queue_Operations."Enqueue") -> ("error out"=w402:errorcluster)  [unwired: 11 in, 1 out]
          }
          frame True {
            w416 = FALSE
            # "Populate the Tree with the measurements"
            n167 = call "Populate Tree.vi"("TreeControl in"=w428, "VI list"=w418, "Folder list"=w417, "error in (no error)"=w431) -> ("TreeControl out"=w425:refnum<vi>, "error out"=w426:errorcluster)  [unwired: 10 in]
            n168 = call "Set Tree Item Icon.vi"("TreeControl in"=w425, "error in (no error)"=w426) -> ("TreeControl out"=w421:refnum<vi>, "Measurement folder Tags"=w419:string[], "Measurement file Tags"=w420:string[], "error out"=w424:errorcluster)  [unwired: 10 in]
            n169 = Empty Array?(array=w420) -> (empty?=w409:bool)
            n170 = Select(t="No Measurement found in the folder" ("Warning"), s=w409, f="Atleast one measurement should be selected" ("Text.Text")) -> (s? t:f=w410:string)
            n171 = property on="Selection warning" class="Str"(error in=w424, "Visible"=TRUE, "Text.Text"=w410) -> (error out=w415:errorcluster)  [unwired: 1 in, 1 out]
            n172 = Select(t=T4."Disabled and Grayed Out" ("Disabled"), s=w409, f=T4."Enabled") -> (s? t:f=w408:T4)
            n173 = Bundle By Name(cluster=w430, "Tree Reference"=w421, "Measurement folder Tags"=w419, "Measurement file Tags"=w420, "Select all"=w416) -> (w429:T3)
            n174 = property on="Select all" class="Bool (strict)"(error in=w415, "Value"=w416, "DisabledEnum"=w408) -> (error out=w422:errorcluster)  [unwired: 1 in, 1 out]
            n175 = property on="Tab Control" class="TabCtl (strict)"(error in=w422, "Value"=T1."Select measurements" ("Tab Control")) -> (error out=w427:errorcluster)  [unwired: 1 in, 1 out]
          }
        }
        n176 = property on="Info" class="Str"(error in=w379, "Visible"=FALSE) -> (error out=w378:errorcluster)  [unwired: 1 in, 1 out]
        n177 = call "Set Cursor Icon.vi"("Cursor icon"=u16 0, "error in (no error)"=w378) -> ("error out"=w388:errorcluster)  [unwired: 13 in]
      }
      frame "Select/Deselect all" {
        # "Update the selection of items in the Tree based on the value of Select all"
        n178 = call "Set Cursor Icon.vi"("Cursor icon"=u16 2, "error in (no error)"=w446) -> ("error out"=w435:errorcluster)  [unwired: 13 in]
        n179 = Unbundle By Name(w438) -> ("Tree Reference"=w439:refnum<vi>, "Measurement folder Tags"=w441:string[], "Measurement file Tags"=w443:string[], "Select all"=w445:bool)
        n180 = Not(x=w445) -> (.not. x?=w447:bool)
        n181 = call "Tree Icons.vi"() -> ("Not Selected"=w449:i32, "Selected"=w450:i32)  [unwired: 6 in]
        n182 = property on="Selection warning" class="Str"(error in=w435, "Text.Text"="Atleast one measurement should be selected", "Visible"=w447) -> (error out=w444:errorcluster)  [unwired: 1 in, 1 out]
        n183 = Select(t=w450, s=w445, f=w449) -> (s? t:f=w442:i32)
        n184 = call "Update Tree Item Icon.vi"("TreeControl in"=w439, "Measurement folder Tags"=w441, "Measurement file Tags"=w443, "Icon"=w442, "error in (no error)"=w444) -> ("TreeControl out"=w436:refnum<vi>, "error out"=w440:errorcluster)  [unwired: 9 in]
        n185 = Bundle By Name(cluster=w438, "Tree Reference"=w436) -> (w437:T3)
        n186 = call "Set Cursor Icon.vi"("Cursor icon"=u16 0, "error in (no error)"=w440) -> ("error out"=w434:errorcluster)  [unwired: 13 in]
      }
      frame "Measurement selection" {
        # "Update the icons of the Tree items based on the selection"
        n187 = call "Set Cursor Icon.vi"("Cursor icon"=u16 2, "error in (no error)"=w471) -> ("error out"=w456:errorcluster)  [unwired: 13 in]
        n188 = Unbundle By Name(w470) -> ("Tree Reference"=w451:refnum<vi>, "Measurement folder Tags"=w461:string[], "Measurement file Tags"=w460:string[], "Selected cell Tag"=w462:string)
        n189 = call "Update Tree Item Selection.vi"("TreeControl in"=w451, "Measurement folder Tags"=w461, "Measurement file Tags"=w460, "Selected cell Tag"=w462, "error in (no error)"=w456) -> ("TreeControl out"=w457:refnum<vi>, "error out"=w467:errorcluster)  [unwired: 9 in]
        n190 = Insert Into Array(array=w461, new element=w460) -> (w463:string[])  [unwired: 1 in]
        n191 = call "Verify Select All.vi"("TreeControl in"=w457, "Measurement Tags"=w463, "error in (no error)"=w467) -> ("TreeControl out"=w459:refnum<vi>, "Select"=w452:bool, "Deselect"=w458:bool, "error out"=w466:errorcluster)  [unwired: 9 in]
        n192 = Bundle By Name(cluster=w470, "Tree Reference"=w459, "Select all"=w452) -> (w469:T3)
        n193 = property on="Select all" class="Bool (strict)"(error in=w466, "Value"=w452) -> (error out=w465:errorcluster)  [unwired: 1 in, 1 out]
        n194 = property on="Selection warning" class="Str"(error in=w465, "Text.Text"="Atleast one measurement should be selected", "Visible"=w458) -> (error out=w468:errorcluster)  [unwired: 1 in, 1 out]
        n195 = call "Set Cursor Icon.vi"("Cursor icon"=u16 0, "error in (no error)"=w468) -> ("error out"=w454:errorcluster)  [unwired: 13 in]
      }
      frame "List plug-ins" {
        # "List the Plug-in names of the selected measurements"
        n196 = Unbundle By Name(w477) -> ("Tree Reference"=w482:refnum<vi>, "Measurement file Tags"=w488:string[], "Measurement folder selected?"=w491:bool, "Measurement file/folder path"=w490:path)
        n197 = call "Set Cursor Icon.vi"("Cursor icon"=u16 2, "error in (no error)"=w492) -> ("error out"=w481:errorcluster)  [unwired: 13 in]
        n198 = case "Measurement Folder?" shown="True" w491 {
          tunnel: w481 -> [w507 w513]
          tunnel: w490 -> [w506 _]
          tunnel: [w505 w510] -> w489
          tunnel: [w503 w509] -> w474
          tunnel: w488 -> [_ w512]
          tunnel: w482 -> [w502 w511]
          tunnel: [w502 w508] -> w475
          frame False {
            # "Get the plug-in name of the selected measurement file"
            n199 = call <vilib>:"Get File Extension.vi"("error in (no error)"=w507, "file"=w506) -> ("error out"=w505:errorcluster, "filename without extension"=w501:string)  [unwired: 5 in, 3 out]
            n200 = Build Array(w501, w501) -> (w504:string[])
            n201 = Build Array(w504) -> (w503:string[][])
          }
          frame True {
            # "Get the plug-in names of all the selected files in the measurement folder"
            n202 = call "Get Selected Measurements.vi"("Tree control in"=w511, "Measurement file Tags"=w512, "error in (no error)"=w513) -> ("Tree control out"=w508:refnum<vi>, "Measurement Plug-ins"=w509:string[][], "error out"=w510:errorcluster)  [unwired: 10 in]
          }
        }
        n203 = Index Array(array=w474, index (col)=0 ("index (row)")) -> (element=w473:string[])  [unwired: 1 in]
        n204 = property on="List of Selected Measurements" class="MCListbox (strict)"(error in=w489, "ItemNames"=w474, "TopLeft"=T5 {"Row"=0, "Column"=0} ("Top Left Visible Cell")) -> (error out=w487:errorcluster)  [unwired: 1 in, 1 out]
        n205 = Bundle By Name(cluster=w477, "Tree Reference"=w475, "Measurement Plug-ins"=w474, "Selected Measurement"=w473) -> (w476:T3)
        n206 = Array Size(array=w474) -> (size(s)=w485:i32[])
        n207 = Index Array(array=w485) -> (element=w484:i32)  [unwired: 1 in]
        n208 = for {
          N: w484 -> [_]
          shift-right: [w498] -> w486
          shift-left: w487 -> [w499]
          i -> [w495]
          # "Set the row size for the occupied rows"
          n209 = Bundle By Name(cluster=T6 {"Row"=0, "Column"=0} ("Active Cell:Active Cell"), "Row"=w495) -> (w497:T6)
          n210 = property on="List of Selected Measurements" class="MCListbox (strict)"(error in=w499, "ActiveCell"=w497, "Height"=u32 18 ("Active Cell:Cell Size:Height")) -> (error out=w498:errorcluster)  [unwired: 1 in, 1 out]
        }
        n211 = property on="Tab Control" class="TabCtl (strict)"(error in=w486, "Value"=T1."List Plug-ins" ("Tab Control")) -> (error out=w494:errorcluster)  [unwired: 1 in, 1 out]
        n212 = call "Set Cursor Icon.vi"("Cursor icon"=u16 0, "error in (no error)"=w494) -> ("error out"=w479:errorcluster)  [unwired: 13 in]
      }
      frame "Validate plug-in rename" {
        # "Validate the name of the Plug-in after rename"
        n213 = call "Set Cursor Icon.vi"("Cursor icon"=u16 2, "error in (no error)"=w549) -> ("error out"=w541:errorcluster)  [unwired: 13 in]
        n214 = property on="List of Selected Measurements" class="MCListbox (strict)"(error in=w541) -> (error out=w533:errorcluster, "ItemNames"=w547:string[][])  [unwired: 1 in, 1 out]
        n215 = Unbundle By Name(w545) -> ("Measurement Plug-ins"=w543:string[][], "Project path"=w531:path)
        n216 = Index Array(array=w547, index (col)=1 ("disabled index (col)")) -> (element=w516:string[])  [unwired: 1 in]
        n217 = call "Get Libraries in Project.vi"("Project path"=w531, "error in (no error)"=w533) -> ("Project exists?"=w530:bool, "Library names"=w529:string[], "error out"=w532:errorcluster)  [unwired: 11 in]
        n218 = Index Array(array=w543, index (col)=1 ("disabled index (col)")) -> (element=w515:string[])  [unwired: 1 in]
        n219 = for {
          shift-right: [w556] -> w526
          shift-left: w532 -> [w557]
          tunnel: w516 -> [w553] mode=indexing
          tunnel: w530 -> [w555]
          tunnel: w529 -> [w554]
          tunnel: [w551] -> w517 mode=indexing
          tunnel: w515 -> [w552] mode=indexing
          tunnel: [w550] -> w514 mode=indexing
          # "Validate the plug-in names"
          n220 = call "Validate Plugin Name.vi"("Project exists?"=w555, "Library names"=w554, "Plug-in name"=w553, "error in (no error)"=w557) -> ("Valid Name?"=w551:bool, "error out"=w556:errorcluster)  [unwired: 10 in]
          n221 = Swap Values(12:w552, 13:w551, 14:w553) -> (1:w550:string)  [unwired: 1 out]
        }
        n222 = call "Set Plug-in Name Warning.vi"("Valid Name?"=w517, "Validated names"=w514, "error in (no error)"=w526) -> ("Warning?"=w527:bool, "error out"=w525:errorcluster)  [unwired: 11 in]
        n223 = Replace Array Subset(array=w543, new element=w514, index (col)=1 ("disabled index (col)")) -> (w518:string[][])  [unwired: 1 in]
        n224 = property on="Plug-in warning" class="Str"(error in=w525, "Visible"=w527) -> (error out=w537:errorcluster)  [unwired: 1 in, 1 out]
        n225 = Swap Values(12:u32 250 ("Size:Height"), 13:w527, 14:210 ("x")) -> (1:w528:u32)  [unwired: 1 out]
        n226 = Bundle By Name(cluster=w545, "Measurement Plug-ins"=w518) -> (w544:T3)
        n227 = property on="List of Selected Measurements" class="MCListbox (strict)"(error in=w537, "ItemNames"=w518, "Height"=w528) -> (error out=w534:errorcluster)  [unwired: 1 in, 1 out]
        n228 = Not(x=w527) -> (.not. x?=w522:bool)
        n229 = property on="Plug-in info" class="Str"(error in=w534, "Visible"=w522) -> (error out=w524:errorcluster)  [unwired: 1 in, 1 out]
        n230 = Select(t=T4."Enabled", s=w522, f=T4."Disabled and Grayed Out" ("Disabled")) -> (s? t:f=w519:T4)
        n231 = property on="Start Migration" class="Bool"(error in=w524, "DisabledEnum"=w519) -> (error out=w523:errorcluster)  [unwired: 1 in, 1 out]
        n232 = call "Set Cursor Icon.vi"("Cursor icon"=u16 0, "error in (no error)"=w523) -> ("error out"=w539:errorcluster)  [unwired: 13 in]
      }
      frame "/**********MULTIPLE MIGRATION**********/" {
      }
      frame "Update Measurement Paths" {
        w573 = 70  # Remaining Progress
        # "Update the measurement file paths for measurement folder"
        n233 = property on="Progress" class="Slide (strict)"(error in=w566, "Value"=5 ("Progress"), "Caption.Text"="Getting paths...") -> (error out=w574:errorcluster)  [unwired: 1 in, 1 out]
        n234 = Unbundle By Name(w579) -> ("Migration Status"=w569:string[][], "Measurement file/folder path"=w582:path, "Measurement Plug-ins"=w581:string[][], "Measurement folder selected?"=w580:bool, "Selected Measurement"=w560:string[])  [unwired: 1 out]
        n235 = property on="Measurement Count" class="Slide (strict)"(error in=w574, "Value"=0 ("Measurement Count"), "Caption.Text"="Updating Measurement Paths") -> (error out=w570:errorcluster)  [unwired: 1 in, 1 out]
        n236 = call "Get Measurement Paths.vi"("Measurement Path"=w582, "Measurement Plug-ins"=w581, "Measurement folder selected?"=w580, "error in"=w570) -> ("Measurement Path Array"=w577:path[], "error out"=w562:errorcluster)  [unwired: 10 in]
        n237 = Insert Into Array(array=w569, index (col)=0 ("disabled index (col)"), new element=w560) -> (w567:string[][])  [unwired: 1 in]
        n238 = Array Size(array=w577) -> (size(s)=w572:i32)
        n239 = Quotient & Remainder(x=w573, y=w572) -> (floor(x/y)=w571:i32)  [unwired: 1 out]
        n240 = Bundle By Name(cluster=w579, "Migration Status"=w567, "Measurement File Paths"=w577, "Plugin Migration Value"=w572, "Progress per measurement"=w571) -> (w578:T3)
        n241 = property on="Progress" class="Slide (strict)"(error in=w562, "Value"=15 ("Progress")) -> (error out=w561:errorcluster)  [unwired: 1 in, 1 out]
      }
      frame "Create Project" {
        # "Check if project exists and creates a new project if not present."
        n242 = property on="Progress" class="Slide (strict)"(error in=w586, "Value"=10 ("Progress"), "Caption.Text"="Checking for project...") -> (error out=w587:errorcluster)  [unwired: 1 in, 1 out]
        n243 = property on="Measurement Count" class="Slide (strict)"(error in=w587, "Value"=10 ("Measurement Count"), "Caption.Text"="Creating project if not exist") -> (error out=w590:errorcluster)  [unwired: 1 in, 1 out]
        n244 = Unbundle By Name(w594) -> ("Project path"=w593:path)
        n245 = call "Create and Save Project.vi"("Project Path"=w593, "error in (no error)"=w590) -> ("error out"=w584:errorcluster)  [unwired: 13 in]
        n246 = property on="Progress" class="Slide (strict)"(error in=w584, "Value"=15 ("Progress")) -> (error out=w583:errorcluster)  [unwired: 1 in, 1 out]
      }
      frame "Migrate measurements" {
        # "Migrate multiple measurements along with their shared dependencies"
        n247 = property on="Progress" class="Slide (strict)"(error in=w596, "Value"=0 ("Progress")) -> (error out=w597:errorcluster)  [unwired: 1 in, 1 out]
        n248 = Unbundle By Name(w607) -> ("Project path"=w611:path, "Measurement File Paths"=w609:path[], "Measurement Plug-ins"=w612:string[][])
        n249 = property on="Measurement Count" class="Slide (strict)"(error in=w597, "Value"=20 ("Measurement Count"), "Caption.Text"="Migrating measurement(s)") -> (error out=w602:errorcluster)  [unwired: 1 in, 1 out]
        n250 = Index Array(array=w612, index (col)=1 ("disabled index (col)")) -> (element=w610:string[])  [unwired: 1 in]
        n251 = control-ref of="Progress"() -> (w595:refnum<vi>)
        n252 = call "Migrate Dependencies.vi"("Project path"=w611, "Measurement paths"=w609, "Plug-in names"=w610, "Progress"=w595, "error in"=w602) -> ("Instrument containing subVIs"=w606:path[][], "error out"=w600:errorcluster)  [unwired: 9 in]
        n253 = Bundle By Name(cluster=w607, "Instrument containing subVIs"=w606, "Measurement Progress"=30) -> (w608:T3)
        n254 = property on="Measurement Count" class="Slide (strict)"(error in=w600, "Value"=30 ("Measurement Count")) -> (error out=w599:errorcluster)  [unwired: 1 in, 1 out]
      }
      frame "Enqueue Migration Steps" {
        # "Enqueue the set of states for measurement migration"
        n255 = Unbundle By Name(w618) -> ("Plugin Migration Value"=w617:i32)
        n256 = Greater Than 0?(x=w617) -> (x > 0?=w616:bool)
        n257 = case shown="True" w616 {
          tunnel: w615 -> [w621 w628]
          tunnel: [w623 w627] -> w614
          frame False {
            # "Enqueue next step if all measurements are migrated"
            n258 = property on="Measurement Count" class="Slide (strict)"(error in=w621, "Value"=100 ("Progress")) -> (error out=w622:errorcluster)  [unwired: 1 in, 1 out]
            n259 = call "Queue Driver.vi"("States[]"=string[] ["Save Project", "Show Next Steps"], "error in (no error)"=w622, "Q Operations"=Queue_Operations."Enqueue N") -> ("error out"=w623:errorcluster)  [unwired: 11 in, 1 out]
          }
          frame True {
            # "Enqueue, if there are measurements yet to migrate"
            n260 = call "Queue Driver.vi"("States[]"=string[] ["Set Values in Dict", "Create Plugin Template", "Get Driver List", "Edit Measurement Configuration", "Edit Measurement Results", "Edit Measurement Connector Pane", "Create Wrapper", "Deserialize Cluster Data", "Add Measurement Plugin APIs", "Disable Initialize APIs", "Edit Type Specialization", "Add UI Elements", "Flatten the Clusters", "Handling Default Value", "Update Migration Count"], "error in (no error)"=w628, "Q Operations"=Queue_Operations."Enqueue N") -> ("error out"=w627:errorcluster)  [unwired: 11 in, 1 out]
          }
        }
      }
      frame "Set Values in Dict" {
        # "Measurement Status Message: Migrating 1 of N measurement(s)"
        # "Set values to the Dictionary APIs"
        n261 = Unbundle By Name(w651) -> ("Project path"=w645:path, "Instrument containing subVIs"=w641:path[][], "Measurement Plug-ins"=w650:string[][], "Migration Count"=w629:i32, "Measurement File Paths"=w638:path[])
        n262 = property on="Progress" class="Slide (strict)"(error in=w632, "Value"=0 ("Progress")) -> (error out=w637:errorcluster)  [unwired: 1 in, 1 out]
        n263 = Array Size(array=w638) -> (size(s)=w630:i32)
        n264 = Increment(x=w629) -> (x+1=w634:i32)
        n265 = Format Into String(format string="Migrating %d of %d measurement(s)", error in=w637, w634, w630) -> (resulting string=w635:string, error out=w636:errorcluster)  [unwired: 1 in]
        n266 = property on="Measurement Count" class="Slide (strict)"(error in=w636, "Caption.Text"=w635) -> (error out=w639:errorcluster)  [unwired: 1 in, 1 out]
        n267 = Index Array(array=w638, index=w629) -> (element=w648:path)
        n268 = call "Set Code Module Path.vi"("CodeModule Path"=w648, "error in (no error)"=w639) -> ("error out"=w647:errorcluster)  [unwired: 13 in]
        n269 = Index Array(array=w650, index (row)=w629, index (col)=1 ("disabled index (col)")) -> (element=w646:string)
        n270 = Index Array(array=w641, index (row)=w629) -> (element=w644:path[])  [unwired: 1 in]
        n271 = call "Set Measurement Name.vi"("Name"=w646, "error in (no error)"=w647) -> ("error out"=w643:errorcluster)  [unwired: 13 in]
        n272 = call "Set Instrument VI Paths.vi"("error in (no error)"=w643, "VI Paths[]"=w644) -> ("error out"=w642:errorcluster)  [unwired: 9 in]
        n273 = call "Set Project Path.vi"("Project Path"=w645, "error in (no error)"=w642) -> ("error out"=w631:errorcluster)  [unwired: 13 in]
      }
      frame "Create Plugin Template" {
        # "Create Measurement Plugin Template"
        n274 = property on="Progress" class="Slide (strict)"(error in=w658, "Value"=1 ("Progress"), "Caption.Text"="Creating G Plugin...") -> (error out=w655:errorcluster)  [unwired: 1 in, 1 out]
        n275 = call "Copy Gplugin datafile.vi"("error in (no error)"=w655) -> ("error out"=w656:errorcluster)  [unwired: 14 in]
        n276 = call "Create PPL.vi"("error in (no error)"=w656) -> ("error out"=w654:errorcluster)  [unwired: 14 in]
        n277 = call "Copy plugin Sdk template.vi"("error in (no error)"=w654) -> ("error out"=w652:errorcluster)  [unwired: 14 in]
        n278 = call "Hide the SessionId.vi"("error in (no error)"=w652) -> ("error out"=w653:errorcluster)  [unwired: 14 in]
      }
      frame "Save Project" {
        # "Saving the project and libraries"
        n279 = property on="Progress" class="Slide (strict)"(error in=w662, "Value"=15 ("Progress"), "Caption.Text"="Saving the project files...") -> (error out=w664:errorcluster)  [unwired: 1 in, 1 out]
        n280 = call "Save Projects and Libraries.vi"("error in (no error)"=w664) -> ("error out"=w663:errorcluster)  [unwired: 10 in]
      }
      frame "Update Migration Count" {
        # "Updating the migration count and migration status"
        n281 = in-place {
          in-place-border: [w675] -> w669
          n282 = in-place-cluster #2(w674) -> ("Plugin Migration Value"=w687:i32, "Migration Count"=w678:i32, "Measurement Progress"=w685:i32, "Progress per measurement"=w684:i32, "Migration Status"=w681:string[][])
          n283 = Index Array(array=w681, index (col)=1 ("disabled index (col)")) -> (element=w679:string[])  [unwired: 1 in]
          n284 = Insert Into Array(array=w679, index=w678, new element="Success") -> (w676:string[])
          n285 = Insert Into Array(array=w681, index (col)=1 ("disabled index (col)"), new element=w676) -> (w683:string[][])  [unwired: 1 in]
          n286 = Increment(x=w678) -> (x+1=w688:i32)
          n287 = Add(x=w685, y=w684) -> (x+y=w675:i32)
          n288 = Decrement(x=w687) -> (x-1=w686:i32)
          n289 = in-place-cluster #2("Plugin Migration Value"=w686, "Migration Count"=w688, "Measurement Progress"=w675, "Progress per measurement"=w684, "Migration Status"=w683) -> (w673:T3)
        }
        n290 = property on="Measurement Count" class="Slide (strict)"(error in=w668, "Value"=w669) -> (error out=w667:errorcluster)  [unwired: 1 in, 1 out]
        n291 = call "Queue Driver.vi"("State"="Enqueue Migration Steps", "error in (no error)"=w667, "Q Operations"=Queue_Operations."Enqueue") -> ("error out"=w672:errorcluster)  [unwired: 11 in, 1 out]
      }
      frame "Update count on Fail" {
        # "Updating the migration count and migration status"
        n292 = in-place {
          in-place-border: [w697] -> w691
          n293 = in-place-cluster #3(w696) -> ("Plugin Migration Value"=w709:i32, "Migration Count"=w700:i32, "Measurement Progress"=w707:i32, "Progress per measurement"=w706:i32, "Migration Status"=w703:string[][])
          n294 = Index Array(array=w703, index (col)=1 ("disabled index (col)")) -> (element=w701:string[])  [unwired: 1 in]
          n295 = Insert Into Array(array=w701, index=w700, new element="Fail") -> (w698:string[])
          n296 = Insert Into Array(array=w703, index (col)=1 ("disabled index (col)"), new element=w698) -> (w705:string[][])  [unwired: 1 in]
          n297 = Increment(x=w700) -> (x+1=w710:i32)
          n298 = Add(x=w707, y=w706) -> (x+y=w697:i32)
          n299 = Decrement(x=w709) -> (x-1=w708:i32)
          n300 = in-place-cluster #3("Plugin Migration Value"=w708, "Migration Count"=w710, "Measurement Progress"=w697, "Progress per measurement"=w706, "Migration Status"=w705) -> (w695:T3)
        }
        n301 = property on="Measurement Count" class="Slide (strict)"(error in=w690, "Value"=w691) -> (error out=w689:errorcluster)  [unwired: 1 in, 1 out]
        n302 = call "Queue Driver.vi"("State"="Enqueue Migration Steps", "error in (no error)"=w689, "Q Operations"=Queue_Operations."Enqueue") -> ("error out"=w694:errorcluster)  [unwired: 11 in, 1 out]
      }
      frame "/**********NEXT STEPS POST MIGRATION**********/" {
      }
      frame "Show Next Steps" {
        # "To change unwanted loading symbol"
        # "Showing the migration status"
        n303 = in-place {
          in-place-border: [w736] -> w720
          n304 = in-place-cluster #4(w728) -> ("Migration Status"=w737:string[][])
          n305 = Index Array(array=w737, index (col) #1=0 ("disabled index (col)"), index (col) #2=1 ("index (col)")) -> (element #1=w740:string[], element #2=w738:string[])  [unwired: 2 in]
          n306 = for {
            tunnel: w740 -> [_] mode=indexing
            tunnel: w738 -> [w747]
            shift-right: [w742] -> w736
            shift-left: w737 -> [w745]
            i -> [w744]
            n307 = Index Array(array=w747, index=w744) -> (element=w746:string)
            n308 = Empty String/Path?(string/path=w746) -> (empty?=w743:bool)
            n309 = case shown="True" w743 {
              tunnel: w745 -> [w748 w755]
              tunnel: w744 -> [_ w752]
              tunnel: [w748 w756] -> w742
              frame False {
              }
              frame True {
                # "Insert 'Fail' for empty status"
                n310 = Index Array(array=w755, index (col)=1 ("disabled index (col)")) -> (element=w753:string[])  [unwired: 1 in]
                n311 = Insert Into Array(array=w753, index=w752, new element="Fail" ("new element/subarray")) -> (w750:string[])
                n312 = Insert Into Array(array=w755, index (col)=1 ("disabled index (col)"), new element=w750) -> (w756:string[][])  [unwired: 1 in]
              }
            }
          }
          n313 = in-place-cluster #4("Migration Status"=w736) -> (w727:T3)
        }
        n314 = property on="Tab Control" class="TabCtl (strict)"(error in=w723, "Value"=T1."Status" ("Tab Control")) -> (error out=w725:errorcluster)  [unwired: 1 in, 1 out]
        n315 = property on="Migration Status" class="MCListbox (strict)"(error in=w725, "Allow Editing Cells"=FALSE) -> (error out=w724:errorcluster)  [unwired: 1 in, 1 out]
        n316 = property on="Migration Status" class="MCListbox (strict)"(error in=w724, "ItemNames"=w720) -> (error out=w715:errorcluster)  [unwired: 1 in, 1 out]
        n317 = Index Array(array=w720, index (col)=1 ("disabled index (col)")) -> (element=w718:string[])  [unwired: 1 in]
        n318 = Equal?(x=w718, y="Fail" ("new element/subarray")) -> (x = y?=w716:bool[])
        n319 = And Array Elements(Boolean array=w716) -> (logical AND=w713:bool)
        n320 = case "All the measurements failed?" shown="True" w713 {
          tunnel: w715 -> [w731 w735]
          tunnel: [w732 w734] -> w714
          frame False {
            n321 = property on="Review" class="Bool"(error in=w731, "BoolText.Text"="Review Plug-ins" ("Boolean Text.Text")) -> (error out=w732:errorcluster)  [unwired: 1 in, 1 out]
          }
          frame True {
            # "Change Bool Text to Start next migration"
            n322 = property on="Review" class="Bool"(error in=w735, "BoolText.Text"="Start Next Migration" ("Boolean Text.Text")) -> (error out=w734:errorcluster)  [unwired: 1 in, 1 out]
          }
        }
        n323 = call "Set Cursor Icon.vi"("Cursor icon"=u16 0, "error in (no error)"=w714) -> ("error out"=w722:errorcluster)  [unwired: 13 in]
      }
      frame "Show Links" {
        # "Showing links for the migrated measurements"
        n324 = Unbundle By Name(w764) -> ("Migration Status"=w766:string[][])
        n325 = for {
          tunnel: w766 -> [w773] mode=indexing
          tunnel: [w767] -> w761 mode=indexing if=w770
          # "Populating combo box with successfully migrated plugin names"
          n326 = Index Array(array=w773, index #1=0 ("index"), index #2=1 ("index")) -> (element #1=w767:string, element #2=w768:string)
          n327 = Equal?(x=w768, y="Success") -> (x = y?=w770:bool)
        }
        n328 = Index Array(array=w761, index=0) -> (element=w757:string)
        n329 = property on="Select Plug-in" class="CmbBox"(error in=w765, "Strings[]"=w761, "Value"=w757) -> (error out=w759:errorcluster)  [unwired: 1 in, 1 out]
        n330 = call "Set Measurement Name.vi"("Name"=w757, "error in (no error)"=w759) -> ("error out"=w758:errorcluster)  [unwired: 13 in]
        n331 = property on="Tab Control" class="TabCtl (strict)"(error in=w758, "Value"=T1."Links" ("Tab Control")) -> (error out=w762:errorcluster)  [unwired: 1 in, 1 out]
      }
      frame "/**********ERROR**********/" {
      }
      frame "Error" {
        # "Handle the error and alert user"
        n332 = call <vilib>:"Clear Errors.vi"("error in (no error)"=w783) -> ("error out"=w784:errorcluster)  [unwired: 5 in, 1 out]
        n333 = Equal?(x=string[] ["Set Values in Dict", "Create Plugin Template", "Get Driver List", "Edit Measurement Configuration", "Edit Measurement Results", "Edit Measurement Connector Pane", "Create Wrapper", "Deserialize Cluster Data", "Add Measurement Plugin APIs", "Disable Initialize APIs", "Edit Type Specialization", "Add UI Elements", "Flatten the Clusters", "Handling Default Value", "Update Migration Count"] ("States[]"), y=w776) -> (x = y?=w778:bool[])
        n334 = call "Queue Driver.vi"("error in (no error)"=w784, "Q Operations"=Queue_Operations."Flush") -> ("error out"=w781:errorcluster)  [unwired: 12 in, 1 out]
        n335 = Or Array Elements(Boolean array=w778) -> (logical OR=w777:bool)
        n336 = case shown="False" w777 {
          tunnel: w781 -> [w791 w803]
          tunnel: [w790 w801] -> w780
          tunnel: w776 -> [w789 _]
          frame False {
            # "If error occurs in other steps"
            n337 = Equal?(x=string[] ["Update Measurement Paths", "Create Project", "Migrate measurements"] ("States[]"), y=w789) -> (x = y?=w787:bool[])
            n338 = Or Array Elements(Boolean array=w787) -> (logical OR=w786:bool)
            n339 = case "Error in Migration?" shown="False" w786 {
              tunnel: w791 -> [w795 w798]
              tunnel: [w794 w797] -> w790
              frame False {
                # "Restart Migration tool"
                n340 = call "Queue Driver.vi"("States[]"=string[] ["Reinitialize", "Initialize UI", "Populate project path"], "error in (no error)"=w795, "Q Operations"=Queue_Operations."Enqueue N") -> ("error out"=w794:errorcluster)  [unwired: 11 in, 1 out]
              }
              frame True {
                # "Show Next steps"
                n341 = call "Queue Driver.vi"("State"="Show Next Steps", "error in (no error)"=w798, "Q Operations"=Queue_Operations."Enqueue") -> ("error out"=w797:errorcluster)  [unwired: 11 in, 1 out]
              }
            }
          }
          frame True {
            # "If error occurs during measurement migration"
            n342 = call "Queue Driver.vi"("State"="Update count on Fail", "error in (no error)"=w803, "Q Operations"=Queue_Operations."Enqueue") -> ("error out"=w801:errorcluster)  [unwired: 11 in, 1 out]
          }
        }
      }
      frame "/**********EXIT**********/" {
      }
      frame "Exit" {
        # "Flush the queue elements and stop execution"
        n343 = call "Queue Driver.vi"("error in (no error)"=w816, "Q Operations"=Queue_Operations."Flush") -> ("error out"=w810:errorcluster)  [unwired: 12 in, 1 out]
        n344 = call "Queue Driver.vi"("error in (no error)"=w810, "Q Operations"=Queue_Operations."Release") -> ("error out"=w809:errorcluster)  [unwired: 12 in, 1 out]
        n345 = Unbundle By Name(w814) -> ("Tree Reference"=w813:refnum<vi>)
        n346 = Close Reference(reference=w813, error in (no error)=w809) -> (error out=w807:errorcluster)
        n347 = call "Dictionary.vi"("error in (no error)"=w807, "Dict States"=Dictionary_States."Delete All") -> ("error out"=w806:errorcluster)  [unwired: 12 in, 1 out]
      }
    }
  }
  n348 = invoke class="VI" method="FP.Close"(error in=w6) -> (error out=→"error out":errorcluster)  [unwired: 2 in, 2 out]
